vi "Remakesb.vi"   [LabVIEW 2015]
uses:
  <vilib>/NXT/Block Support/NXT_InputPort.ctl
  <vilib>/NXT/Block Support/NXT_OutputPort.ctl
  <vilib>/NXT/Dual Mode Library/Sensors/Light_On.vi
  <vilib>/NXT/Dual Mode Library/Sensors/Sonar_cm.vi
  <vilib>/NXT/NXTIO Xnodes/NXTIONodeSubVIs/NXTMoveMotors.vi
  <vilib>/NXT/Dual Mode Library/Waits/Wait_Num(msec).vi
  <vilib>/NXT/NXTIO Xnodes/AddressXNode/NXTIOAddress.xnode
  <vilib>/NXT/Subs/LVHSConnector.ctl
  <vilib>/NXT/NXTIO Xnodes/NXTIOXNode/NXTIO.xnode
  <vilib>/NXT/LegoClasses/BrickReference/BrickReference.lvclass
types:
  T1 = typedef "NXT_OutputPort.ctl" = u8
  T2 = typedef "NXT_InputPort.ctl" = u32
  T3 = typedef "LVHSConnector.ctl" = refnum<class "BrickReference.lvclass">
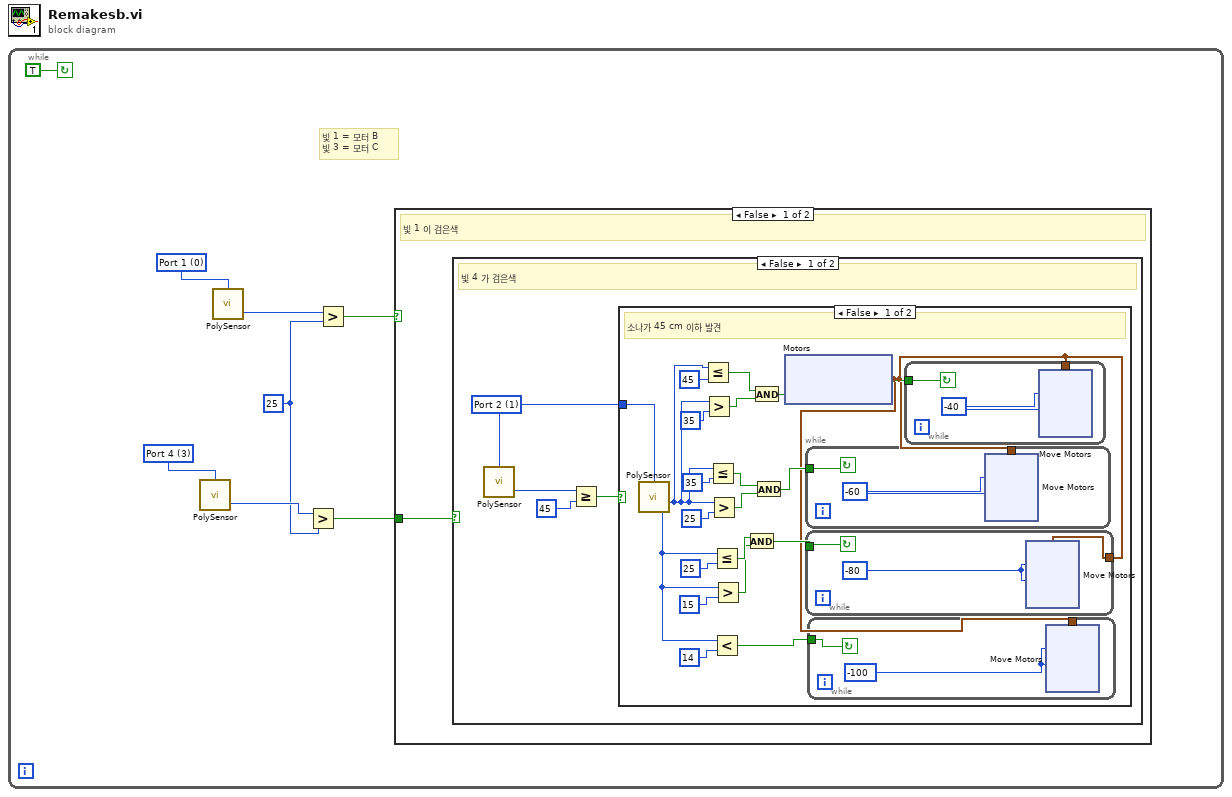
[diagram p0: block diagram]
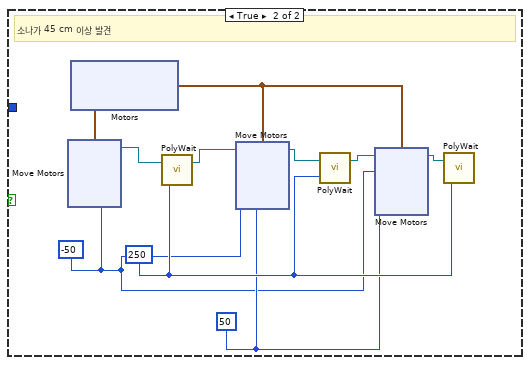
[diagram p2: hidden frame]
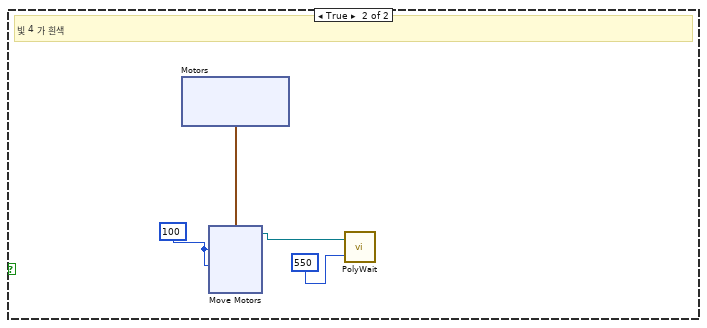
[diagram p3: hidden frame]
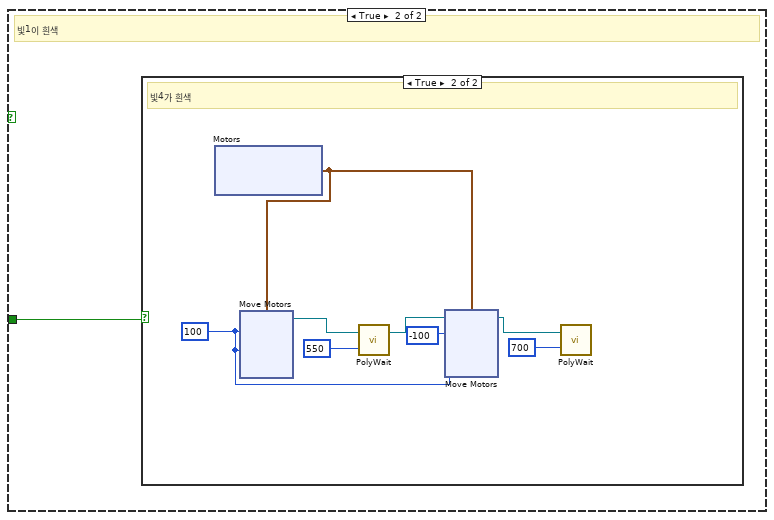
[diagram p4: hidden frame]
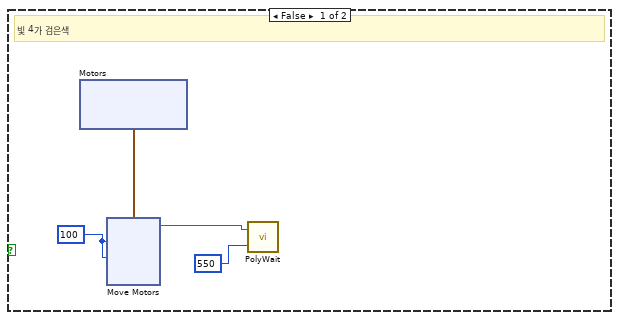
[diagram p5: hidden frame]
diagram:
  n1 = while {
    stop <- TRUE continue-if-true
    w1 = i16 25 ("y")
    w6 = T2 0 items=["Port 1", "Port 2", "Port 3", "Port 4"] ("Port (Port 3)")
    w5 = T2 3 items=["Port 1", "Port 2", "Port 3", "Port 4"] ("Port (Port 3)")
    # "빛 1 = 모터 B\n빛 3 = 모터 C"
    n2 = call-poly <vilib>:"PolySensor.vi"("Port (Port 3)"=w5) -> ("Scaled Value"=w7:i16)  [unwired: 2 in, 1 out]
    n3 = call-poly <vilib>:"PolySensor.vi"("Port (Port 3)"=w6) -> ("Scaled Value"=w8:i16)  [unwired: 2 in, 1 out]
    n4 = Greater?(x=w7, y=w1) -> (0:w3:bool)
    n5 = Greater?(x=w8, y=w1) -> (0:w4:bool)
    n6 = case shown="False" w4 {
      tunnel: w3 -> [w9 w126]
      frame False {
        # "빛 1 이 검은색"
        n7 = case shown="False" w9 {
          frame False {
            w10 = T2 1 items=["Port 1", "Port 2", "Port 3", "Port 4"] ("Port (Port 4)")
            # "빛 4 가 검은색"
            n8 = call-poly <vilib>:"PolySensor.vi"("Port (Port 4)"=w10) -> ("Distance (cm)"=w13:i16)  [unwired: 2 in, 1 out]
            n9 = Greater Or Equal?(x=w13, y=i16 45) -> (x >= y?=w11:bool)
            n10 = case shown="False" w11 {
              tunnel: w10 -> [w33 _]
              frame False {
                # "소나가 45 cm 이하 발견"
                n11 = call-poly <vilib>:"PolySensor.vi"("Port (Port 4)"=w33) -> ("Distance (cm)"=w16:i16)  [unwired: 2 in, 1 out]
                n12 = Less Or Equal?(x=w16, y=i16 45) -> (x <= y?=w30:bool)
                n13 = Greater?(x=w16, y=i16 35) -> (0:w29:bool)
                n14 = Less Or Equal?(x=w16, y=i16 35) -> (x <= y?=w25:bool)
                n15 = Greater?(x=w16, y=i16 25) -> (0:w24:bool)
                n16 = Less Or Equal?(x=w16, y=i16 25) -> (x <= y?=w22:bool)
                n17 = Less?(x=w16, y=i16 14) -> (x < y?=w15:bool)
                n18 = Greater?(x=w16, y=i16 15) -> (0:w21:bool)
                n19 = And(x=w22, y=w21) -> (x .and. y?=w18:bool)
                n20 = And(x=w30, y=w29) -> (x .and. y?=w28:bool)
                n21 = And(x=w25, y=w24) -> (x .and. y?=w23:bool)
                n22 = xnode "Motors"() -> ("Motor"=w14:cluster{"Port":T1, "Port":T1})
                n23 = while {
                  tunnel: w23 -> [w58]
                  tunnel: w14 -> [w57]
                  stop <- w58 continue-if-true
                  w56 = -60
                  n24 = xnode "Move Motors"("Power/Speed 2"=w56, "Power/Speed 1"=w56, "Motors"=w57) -> ()  [unwired: 1 in, 1 out]
                }
                n25 = while {
                  tunnel: w18 -> [w47]
                  tunnel: w14 -> [w46]
                  stop <- w47 continue-if-true
                  w45 = -80
                  n26 = xnode "Move Motors"("Power/Speed 2"=w45, "Power/Speed 1"=w45, "Motors"=w46) -> ()  [unwired: 1 in, 1 out]
                }
                n27 = while {
                  tunnel: w15 -> [w36]
                  tunnel: w14 -> [w35]
                  stop <- w36 continue-if-true
                  w34 = -100
                  n28 = xnode "Move Motors"("Power/Speed 2"=w34, "Power/Speed 1"=w34, "Motors"=w35) -> ()  [unwired: 1 in, 1 out]
                }
                n29 = while {
                  tunnel: w28 -> [w69]
                  tunnel: w14 -> [w68]
                  stop <- w69 continue-if-true
                  w67 = -40
                  n30 = xnode "Move Motors"("Power/Speed 2"=w67, "Power/Speed 1"=w67, "Motors"=w68) -> ()  [unwired: 1 in, 1 out]
                }
              }
              frame True {
                w86 = i16 250 ("y")
                w85 = i16 50 ("y")
                w84 = i16 -50 ("y")
                # "소나가 45 cm 이상 발견"
                n31 = xnode "Motors"() -> ("Motor"=w87:cluster{"Port":T1, "Port":T1})
                n32 = xnode "Move Motors"("Power/Speed 2"=w84, "Power/Speed 1"=w84, "Motors"=w87) -> ("NXT/EV3"=w83:T3)  [unwired: 1 in]
                n33 = call-poly <vilib>:"PolyWait.vi"("Time (100 msec)"=w86, "NXT/EV3"=w83) -> ("NXT/EV3"=w82:T3)  [unwired: 2 in]
                n34 = xnode "Move Motors"("Power/Speed 2"=w84, "Power/Speed 1"=w85, "Motors"=w87, "NXT/EV3"=w82) -> ("NXT/EV3"=w81:T3)
                n35 = call-poly <vilib>:"PolyWait.vi"("Time (100 msec)"=w86, "NXT/EV3"=w81) -> ("NXT/EV3"=w80:T3)  [unwired: 2 in]
                n36 = xnode "Move Motors"("Power/Speed 2"=w85, "Power/Speed 1"=w84, "Motors"=w87, "NXT/EV3"=w80) -> ("NXT/EV3"=w79:T3)
                n37 = call-poly <vilib>:"PolyWait.vi"("Time (100 msec)"=w86, "NXT/EV3"=w79) -> ()  [unwired: 2 in, 1 out]
              }
            }
          }
          frame True {
            w113 = i16 100 ("y")
            # "빛 4 가 흰색"
            n38 = xnode "Motors"() -> ("Motor"=w116:cluster{"Port":T1, "Port":T1})
            n39 = xnode "Move Motors"("Power/Speed 2"=w113, "Power/Speed 1"=w113, "Motors"=w116) -> ("NXT/EV3"=w114:T3)  [unwired: 1 in]
            n40 = call-poly <vilib>:"PolyWait.vi"("Time (100 msec)"=i16 550 ("y"), "NXT/EV3"=w114) -> ()  [unwired: 2 in, 1 out]
          }
        }
      }
      frame True {
        # "빛1이 흰색"
        n41 = case shown="True" w126 {
          frame False {
            w127 = i16 100 ("y")
            # "빛 4가 검은색"
            n42 = xnode "Motors"() -> ("Motor"=w130:cluster{"Port":T1, "Port":T1})
            n43 = xnode "Move Motors"("Power/Speed 2"=w127, "Power/Speed 1"=w127, "Motors"=w130) -> ("NXT/EV3"=w128:T3)  [unwired: 1 in]
            n44 = call-poly <vilib>:"PolyWait.vi"("Time (100 msec)"=i16 550 ("y"), "NXT/EV3"=w128) -> ()  [unwired: 2 in, 1 out]
          }
          frame True {
            w140 = i16 100 ("y")
            # "빛4가 흰색"
            n45 = xnode "Motors"() -> ("Motor"=w147:cluster{"Port":T1, "Port":T1})
            n46 = xnode "Move Motors"("Power/Speed 2"=w140, "Power/Speed 1"=w140, "Motors"=w147) -> ("NXT/EV3"=w146:T3)  [unwired: 1 in]
            n47 = call-poly <vilib>:"PolyWait.vi"("Time (100 msec)"=i16 550 ("y"), "NXT/EV3"=w146) -> ("NXT/EV3"=w145:T3)  [unwired: 2 in]
            n48 = xnode "Move Motors"("Power/Speed 2"=w140, "Power/Speed 1"=i16 -100 ("y"), "Motors"=w147, "NXT/EV3"=w145) -> ("NXT/EV3"=w144:T3)
            n49 = call-poly <vilib>:"PolyWait.vi"("Time (100 msec)"=i16 700 ("y"), "NXT/EV3"=w144) -> ()  [unwired: 2 in, 1 out]
          }
        }
      }
    }
  }
